vi "USB2XXXSPIADS1256.vi"() -> ()   [LabVIEW 2010]
uses:
  PublicFiles/USB2XXX.dll
panel:
  out "mVp-p":dbl
  out "DC":dbl
  out "RMS":dbl
  out "Waveform Chart":dbl(graph)
  in  "pConfig":T1
  in  "Channel Index":i32(ring) items=["SPI1_CS0", "SPI2_CS0"]
  in  "Device Index":i32(ring) items=["0", "1", "2", "3", "4", "5"]
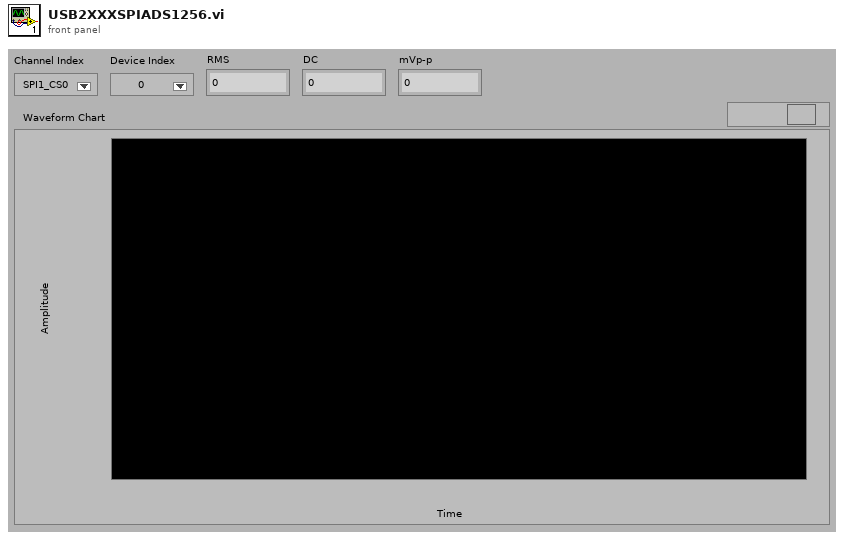
[diagram p1: front panel]
types:
  T1 = cluster{"Mode":i8, "Master":i8, "CPOL":i8, "CPHA":i8, "LSBFirst":i8, "SelPolarity":i8, "@dummy control@":i8, "@dummy control@":i8, "ClockSpeedHz":u32}
  T2 = enum16{"Init ADS1256", "Init SPI", "Read Data", "Close"}
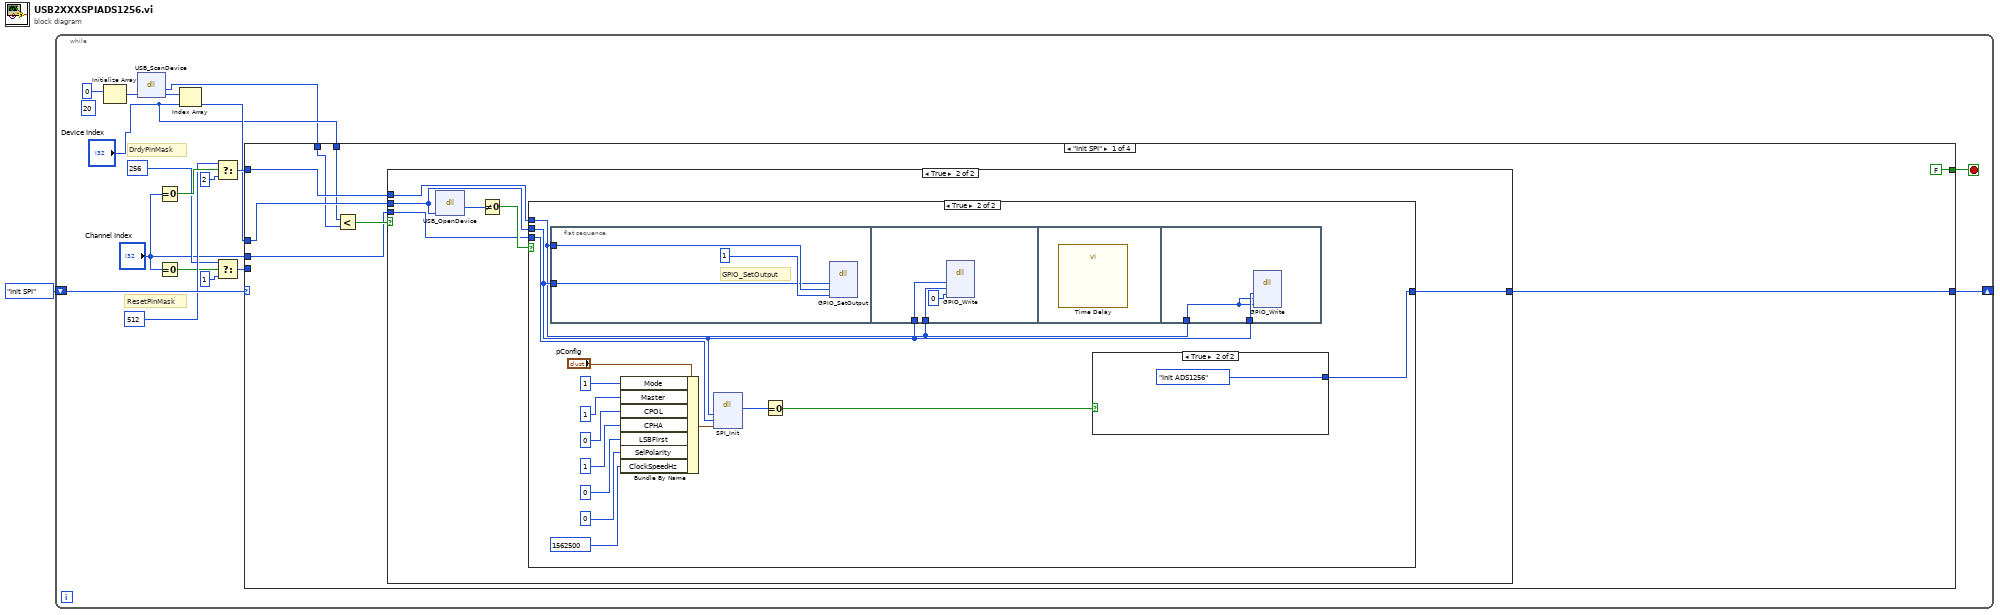
[diagram p0: block diagram]
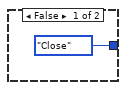
[diagram p2: hidden frame]
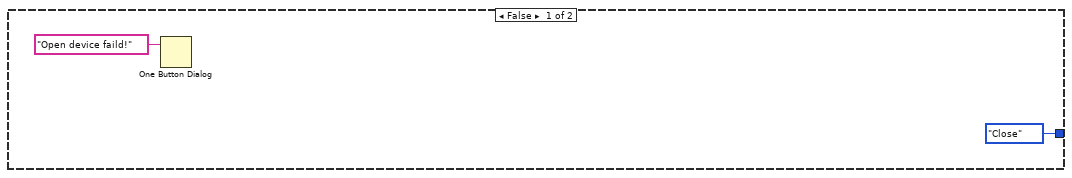
[diagram p3: hidden frame]
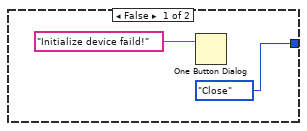
[diagram p4: hidden frame]
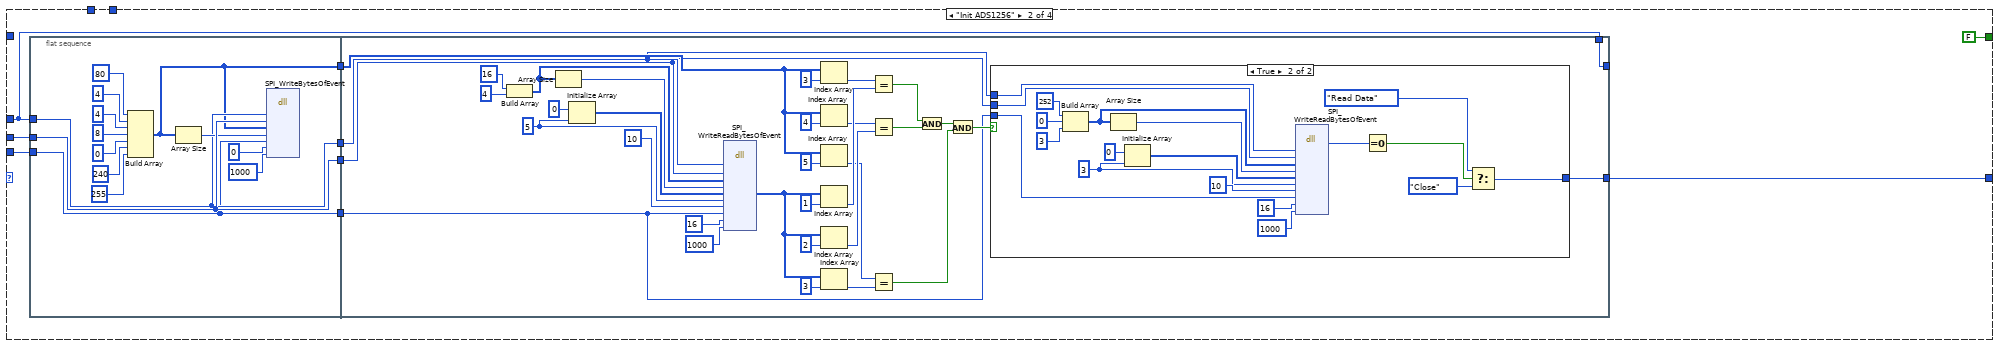
[diagram p5: hidden frame]
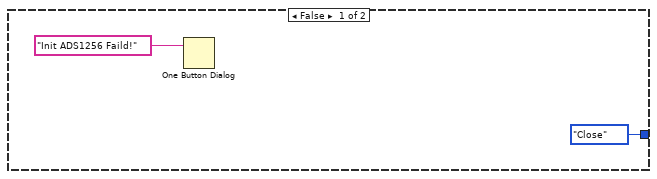
[diagram p6: hidden frame]
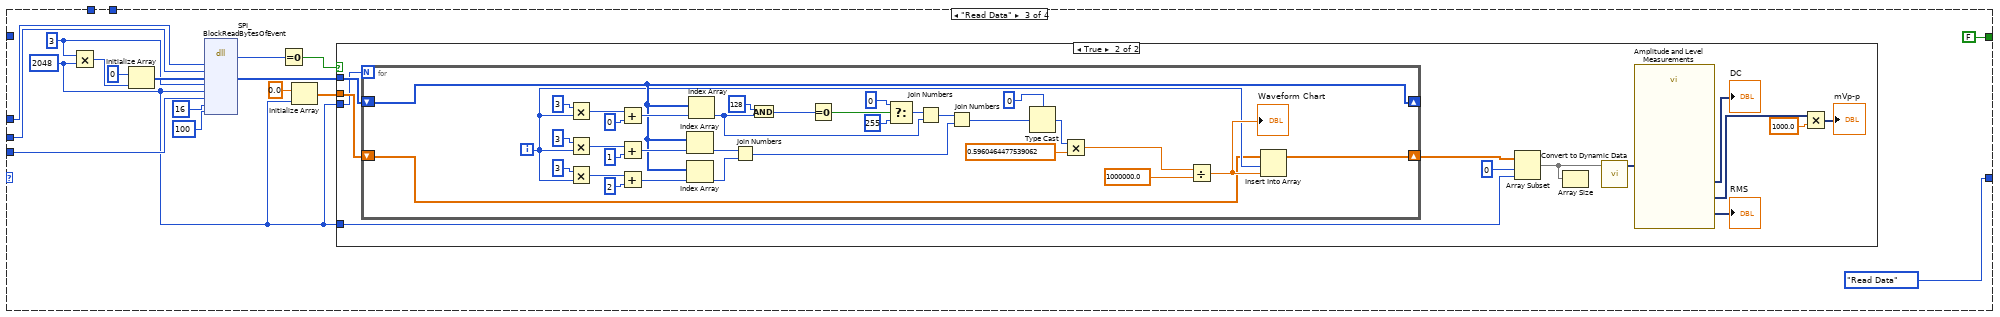
[diagram p7: hidden frame]
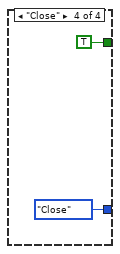
[diagram p9: hidden frame]
diagram:
  n1 = while {
    shift-right: [w18] -> _
    shift-left: T2."Init SPI" ("Enum") -> [w19]
    stop <- w17 stop-if-true
    (unwired) 20 ("dimension size")
    # "DrdyPinMask"
    # "ResetPinMask"
    n2 = Initialize Array(0) -> (w7:i32[])  [unwired: 1 in]
    n3 = dll-call lib="G:/OtherWork/USB2XXX_Example/trunk/Labview/PublicFiles/USB2XXX.*" fn="USB_ScanDevice"("pDevNum"=w7) -> ("return type"=w2:i32, "pDevNum"=w5:i32[])  [unwired: 3 in, 2 out]
    n4 = Equal To 0?(x="Channel Index") -> (x = 0?=w16:bool)
    n5 = Equal To 0?(x="Channel Index") -> (x = 0?=w13:bool)
    n6 = Index Array(array=w5, index="Device Index") -> (element=w4:i32)
    n7 = Select(t=u32 512 ("SelPolarity"), s=w16, f=u32 2 ("SelPolarity")) -> (s? t:f=w9:u32)
    n8 = Select(t=u32 256 ("SelPolarity"), s=w13, f=u32 1 ("SelPolarity")) -> (s? t:f=w8:u32)
    n9 = case shown="\"Init SPI\"" w19 {
      tunnel: [w26 w63 T2."Read Data" ("Enum") T2."Close" ("Enum")] -> w18
      tunnel: w4 -> [w23 w68 w154 _]
      tunnel: "Channel Index" -> [w25 w70 w153 _]
      tunnel: [FALSE FALSE FALSE TRUE] -> w17
      tunnel: w9 -> [w22 _ _ _]
      tunnel: w8 -> [_ w67 w149 _]
      tunnel: w2 -> [w21 _ _ _]
      tunnel: "Device Index" -> [w20 _ _ _]
      frame "Init SPI" {
        n10 = Less?(x=w20, y=w21) -> (x < y?=w27:bool)
        n11 = case shown="True" w27 {
          tunnel: w23 -> [_ w30]
          tunnel: w25 -> [_ w32]
          tunnel: [T2."Close" ("Enum") w31] -> w26
          tunnel: w22 -> [_ w29]
          frame False {
          }
          frame True {
            n12 = dll-call lib="G:/OtherWork/USB2XXX_Example/trunk/Labview/PublicFiles/USB2XXX.*" fn="USB_OpenDevice"("DevIndex"=w30) -> (w34:u8)  [unwired: 4 in, 2 out]
            n13 = Not Equal To 0?(x=w34) -> (x != 0?=w33:bool)
            n14 = case shown="True" w33 {
              tunnel: w32 -> [_ w39]
              tunnel: w30 -> [_ w38]
              tunnel: [T2."Close" ("Enum") w50] -> w31
              tunnel: w29 -> [_ w37]
              frame False {
                n15 = One Button Dialog(message="Open device faild!") -> ()  [unwired: 1 in, 1 out]
              }
              frame True {
                n16 = flat-sequence {
                  tunnel: w37 -> [w53]
                  tunnel: w38 -> [w52]
                  tunnel: w38 -> [w57]
                  tunnel: w37 -> [w56]
                  tunnel: w38 -> [w59]
                  tunnel: w37 -> [w58]
                  frame #0 {
                    # "GPIO_SetOutput"
                    n17 = dll-call lib="G:/OtherWork/USB2XXX_Example/trunk/Labview/PublicFiles/USB2XXX.*" fn="GPIO_SetOutput"("DevIndex"=w52, "PinMask"=w53, "PuPd"=u8 1) -> ()  [unwired: 7 in, 2 out]
                  }
                  frame #1 {
                    n18 = dll-call lib="G:/OtherWork/USB2XXX_Example/trunk/Labview/PublicFiles/USB2XXX.*" fn="GPIO_Write"("DevIndex"=w57, "PinMask"=w56, "PinValue"=u32 0) -> ()  [unwired: 7 in, 2 out]
                  }
                  frame #2 {
                    n19 = call "Time Delay"() -> ()  [unwired: 11 in, 1 out]
                  }
                  frame #3 {
                    n20 = dll-call lib="G:/OtherWork/USB2XXX_Example/trunk/Labview/PublicFiles/USB2XXX.*" fn="GPIO_Write"("DevIndex"=w59, "PinMask"=w58, "PinValue"=w58) -> ()  [unwired: 7 in, 2 out]
                  }
                }
                n21 = Bundle By Name(cluster="pConfig", "Mode"=i8 1, "Master"=i8 1, "CPOL"=i8 0, "CPHA"=i8 1, "LSBFirst"=i8 0, "SelPolarity"=i8 0, "ClockSpeedHz"=u32 1562500) -> (w49:T1)
                n22 = dll-call lib="G:/OtherWork/USB2XXX_Example/trunk/Labview/PublicFiles/USB2XXX.*" fn="SPI_Init"("DevIndex"=w38, "SPIIndex"=w39, "pConfig"=w49) -> (w48:i32)  [unwired: 6 in, 2 out]
                n23 = Equal To 0?(x=w48) -> (x = 0?=w51:bool)
                n24 = case shown="True" w51 {
                  tunnel: [T2."Close" ("Enum") T2."Init ADS1256" ("Enum")] -> w50
                  frame False {
                    n25 = One Button Dialog(message="Initialize device faild!") -> ()  [unwired: 1 in, 1 out]
                  }
                  frame True {
                  }
                }
              }
            }
          }
        }
      }
      frame "Init ADS1256" {
        n26 = flat-sequence {
          tunnel: w68 -> [w74]
          tunnel: w70 -> [w78]
          tunnel: [w78] -> w69
          tunnel: w67 -> [w73]
          tunnel: [w74] -> w66
          tunnel: [w73] -> w65
          tunnel: [w72] -> w64
          tunnel: w69 -> [w87]
          tunnel: [w119] -> _
          tunnel: w68 -> [w119]
          tunnel: w66 -> [w88]
          tunnel: w65 -> [w86]
          tunnel: w64 -> [w101]
          tunnel: [w89] -> w63
          frame #0 {
            n27 = Build Array(u8 80, u8 4, u8 4, u8 8, u8 0, u8 240, u8 255) -> (w72:u8[])
            n28 = Array Size(array=w72) -> (size(s)=w77:i32)
            n29 = dll-call lib="G:/OtherWork/USB2XXX_Example/trunk/Labview/PublicFiles/USB2XXX.*" fn="SPI_WriteBytesOfEvent"("DevIndex"=w74, "SPIIndex"=w78, "pWriteData"=w72, "WriteLen"=w77, "EventPin"=w73, "EventType"=u8 0, "TimeOutOfMs"=1000) -> ()  [unwired: 11 in, 2 out]
          }
          frame #1 {
            w112 = 5 ("dimension size")
            n30 = Build Array(u8 16, u8 4) -> (w115:u8[])
            n31 = Array Size(array=w115) -> (size(s)=w114:i32)
            n32 = Initialize Array(u8 0 ("element"), w112) -> (w113:u8[])
            n33 = dll-call lib="G:/OtherWork/USB2XXX_Example/trunk/Labview/PublicFiles/USB2XXX.*" fn="SPI_WriteReadBytesOfEvent"("DevIndex"=w88, "SPIIndex"=w87, "pWriteData"=w115, "WriteLen"=w114, "pReadData"=w113, "ReadLen"=w112, "IntervalTimeUs"=10, "EventPin"=w86, "EventType"=u8 16, "TimeOutOfMs"=1000) -> ("pReadData"=w102:u8[])  [unwired: 13 in, 2 out]
            n34 = Index Array(array=w101, index=3) -> (element=w100:u8)
            n35 = Index Array(array=w101, index=4) -> (element=w98:u8)
            n36 = Index Array(array=w101, index=5) -> (element=w96:u8)
            n37 = Index Array(array=w102, index=1) -> (element=w99:u8)
            n38 = Index Array(array=w102, index=2) -> (element=w97:u8)
            n39 = Index Array(array=w102, index=3) -> (element=w95:u8)
            n40 = Equal?(x=w100, y=w99) -> (x = y?=w94:bool)
            n41 = Equal?(x=w98, y=w97) -> (x = y?=w93:bool)
            n42 = Equal?(x=w96, y=w95) -> (x = y?=w91:bool)
            n43 = And(x=w94, y=w93) -> (x .and. y?=w92:bool)
            n44 = And(x=w92, y=w91) -> (x .and. y?=w90:bool)
            n45 = case shown="True" w90 {
              tunnel: [T2."Close" ("Enum") w123] -> w89
              tunnel: w88 -> [_ w140]
              tunnel: w87 -> [_ w139]
              tunnel: w86 -> [_ w130]
              frame False {
                n46 = One Button Dialog(message="Init ADS1256 Faild!") -> ()  [unwired: 1 in, 1 out]
              }
              frame True {
                w122 = 3 ("dimension size")
                n47 = Build Array(u8 252, u8 0, u8 3) -> (w135:u8[])
                n48 = Array Size(array=w135) -> (size(s)=w134:i32)
                n49 = Initialize Array(u8 0 ("element"), w122) -> (w132:u8[])
                n50 = dll-call lib="G:/OtherWork/USB2XXX_Example/trunk/Labview/PublicFiles/USB2XXX.*" fn="SPI_WriteReadBytesOfEvent"("DevIndex"=w140, "SPIIndex"=w139, "pWriteData"=w135, "WriteLen"=w134, "pReadData"=w132, "ReadLen"=w122, "IntervalTimeUs"=10, "EventPin"=w130, "EventType"=u8 16, "TimeOutOfMs"=1000) -> (w127:i32)  [unwired: 13 in, 2 out]
                n51 = Equal To 0?(x=w127) -> (x = 0?=w126:bool)
                n52 = Select(t=T2."Read Data" ("Enum"), s=w126, f=T2."Close" ("Enum")) -> (s? t:f=w123:T2)
              }
            }
          }
        }
      }
      frame "Read Data" {
        w141 = 2048 ("element")
        w150 = 3 ("element")
        n53 = Multiply(x=w150, y=w141) -> (x*y=w152:i32)
        n54 = Initialize Array(u8 0 ("element"), w152) -> (w151:u8[])
        n55 = dll-call lib="G:/OtherWork/USB2XXX_Example/trunk/Labview/PublicFiles/USB2XXX.*" fn="SPI_BlockReadBytesOfEvent"("DevIndex"=w154, "SPIIndex"=w153, "pReadData"=w151, "BlockSize"=w150, "BlockNum"=w141, "EventPin"=w149, "EventType"=u8 16, "TimeOutOfMs"=100 ("TimeOutMs")) -> (w146:i32, "pReadData"=w144:u8[])  [unwired: 10 in, 2 out]
        n56 = Equal To 0?(x=w146) -> (x = 0?=w145:bool)
        n57 = Initialize Array(0.0 ("element"), w141) -> (w142:dbl[])
        n58 = case shown="True" w145 {
          tunnel: w141 -> [_ w165]
          tunnel: w144 -> [_ w170]
          tunnel: w142 -> [_ w166]
          tunnel: w141 -> [_ w161]
          frame False {
          }
          frame True {
            n59 = for {
              N: w165 -> [_]
              shift-right: [w175] -> _
              shift-left: w170 -> [w175]
              shift-right: [w171] -> w164
              shift-left: w166 -> [w172]
              i -> [w173]
              n60 = Multiply(x=3 ("element"), y=w173) -> (x*y=w203:i32)
              n61 = Multiply(x=3 ("element"), y=w173) -> (x*y=w198:i32)
              n62 = Multiply(x=3 ("element"), y=w173) -> (x*y=w195:i32)
              n63 = Add(x=w203, y=0) -> (x+y=w201:i32)
              n64 = Add(x=w198, y=1) -> (x+y=w200:i32)
              n65 = Add(x=w195, y=2) -> (x+y=w193:i32)
              n66 = Index Array(array=w175, index=w200) -> (element=w191:u8)
              n67 = Index Array(array=w175, index=w193) -> (element=w192:u8)
              n68 = Index Array(array=w175, index=w201) -> (element=w190:u8)
              n69 = Join Numbers(hi=w191, lo=w192) -> ((hi.lo)=w182:u16)
              n70 = And(x=u8 128 ("element"), y=w190) -> (x .and. y?=w187:u8)
              n71 = Equal To 0?(x=w187) -> (x = 0?=w188:bool)
              n72 = Select(t=u8 0 ("element"), s=w188, f=u8 255 ("element")) -> (s? t:f=w184:u8)
              n73 = Join Numbers(hi=w184, lo=w190) -> ((hi.lo)=w183:u16)
              n74 = Join Numbers(hi=w183, lo=w182) -> ((hi.lo)=w181:u32)
              n75 = Type Cast(type=0 ("element"), x=w181) -> (*(type *) &x=w179:i32)
              n76 = Multiply(x=w179, y=0.5960464477539062) -> (x*y=w177:dbl)
              n77 = Divide(x=w177, y=1000000.0) -> (x/y=w174:dbl)
              "Waveform Chart" <- w174
              n78 = Insert Into Array(array=w172, index=w173, new element=w174) -> (w171:dbl[])
            }
            n79 = Array Subset(array=w164, index=0, length=w161) -> (w163:dbl[])
            n80 = Array Size(array=w163) -> ()  [unwired: 1 out]
            n81 = call "Convert to Dynamic Data"("Array"=w163) -> ("Dynamic Data Type"=w169:dynamicdata)  [unwired: 3 in]
            n82 = call "Amplitude and Level Measurements"("Signals"=w169) -> ("Mean (DC)"=→"DC":dynamicdata, "RMS"=→"RMS":dynamicdata, "Peak to Peak"=w160:dynamicdata)  [unwired: 11 in, 1 out]
            n83 = Multiply(x=w160, y=1000.0) -> (x*y=→"mVp-p":dynamicdata)
          }
        }
      }
      frame "Close" {
      }
    }
  }
